vi "myfirst2.vi"() -> ()   [LabVIEW 2020]
panel:
  in  "Boolean 3":bool
  out "Boolean 2":bool
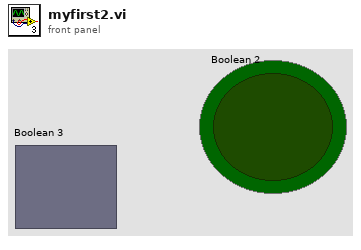
[diagram p1: front panel]
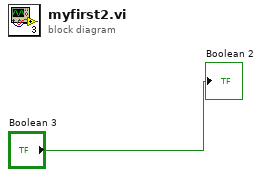
[diagram p0: block diagram]
diagram:
  "Boolean 2" <- "Boolean 3"
